vi "Read Serial Data.vi"(8 "Error In":errorcluster, 11 "VISA Resource In":refnum<visa-resource-name>) -> (0 "Error Out":errorcluster, 2 "Data String":string, 3 "VISA Resource Out":refnum<visa-resource-name>)   [LabVIEW 2013]
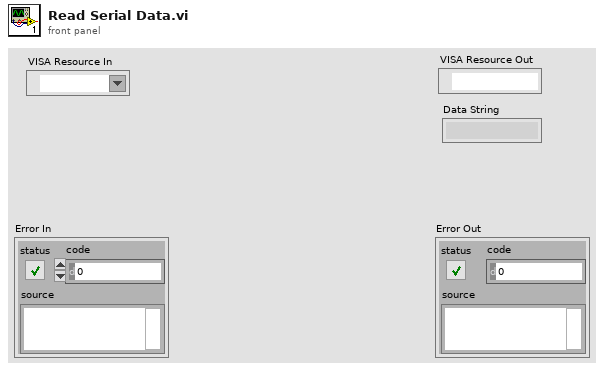
[diagram p1: front panel]
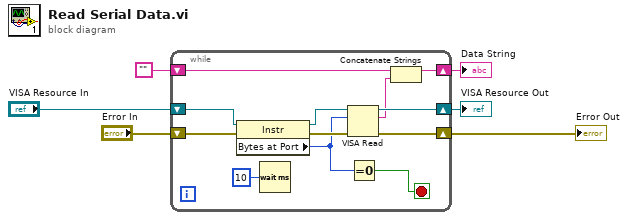
[diagram p0: block diagram]
diagram:
  n1 = while {
    shift-right: [w14] -> w2
    shift-left: "VISA Resource In" -> [w16]
    shift-right: [w13] -> w1
    shift-left: "Error In" -> [w18]
    shift-right: [w9] -> w3
    shift-left: "" -> [w10]
    stop <- w11 stop-if-true
    n2 = property class="Instr"(reference=w16, error in=w18) -> (reference out=w15:refnum<visa-resource-name>, error out=w17:errorcluster, "Bytes at Port"=w12:u32)
    n3 = Wait (ms)(milliseconds to wait=u32 10) -> ()  [unwired: 1 out]
    n4 = VISA Read(VISA resource name=w15, byte count=w12, error in (no error)=w17) -> (VISA resource name out=w14:refnum<visa-resource-name>, read buffer=w8:string, error out=w13:errorcluster)  [unwired: 1 out]
    n5 = Equal To 0?(x=w12) -> (x = 0?=w11:bool)
    n6 = Concatenate Strings(w10, w8) -> (w9:string)
  }
  "Data String" <- w3
  "VISA Resource Out" <- w2
  "Error Out" <- w1
